vi "_PC_SaveFile exportDocData.vi"(7 "xy graph ref":refnum<vi>, 8 "error in (no error)":errorcluster) -> (0 "error out":errorcluster)   [LabVIEW 2018]
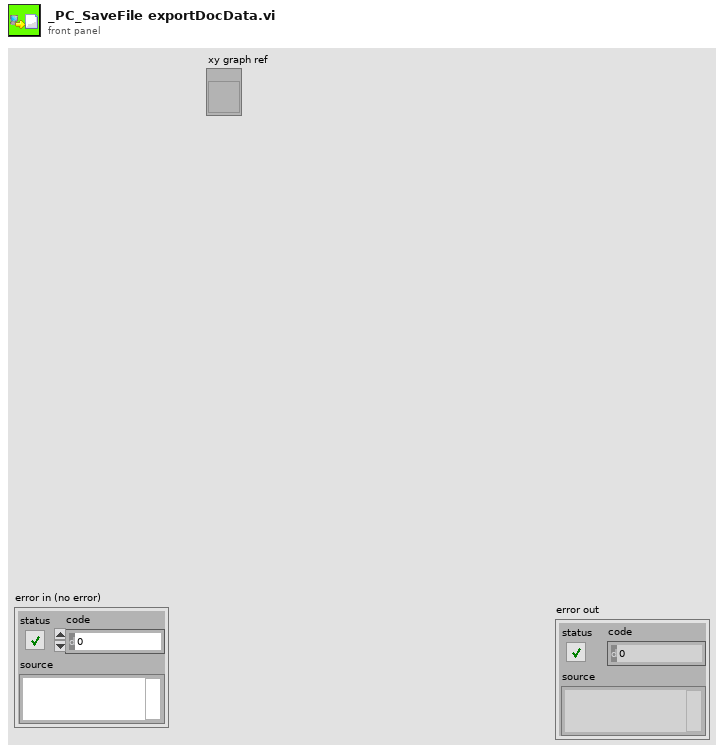
[diagram p1: front panel]
types:
  T1 = enum16{"open", "replace", "create", "open or create", "replace or create", "replace or create with confirmation"}
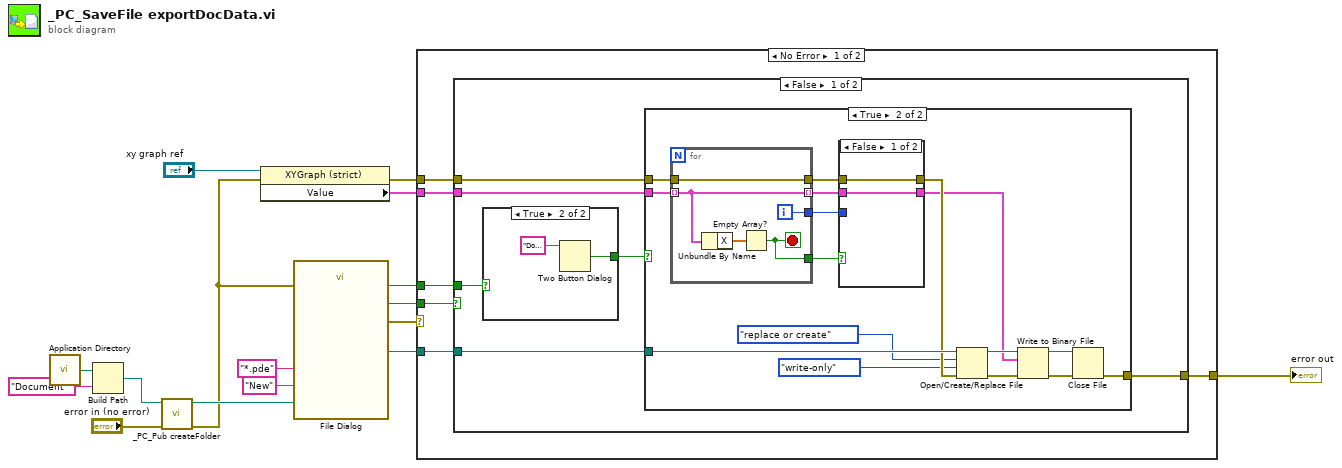
[diagram p0: block diagram]
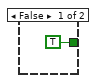
[diagram p2: hidden frame]
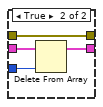
[diagram p4: hidden frame]
diagram:
  n1 = call <vilib>:"Application Directory.vi"() -> ("Application Directory"=w10:path)
  n2 = Build Path(base path=w10, name or relative path="Document") -> (appended path=w4:path)
  n3 = call "_PC_Pub createFolder.vi"("error in (no error)"="error in (no error)", "path (use dialog)"=w4) -> ("error out"=w1:errorcluster, "created path"=w2:path)  [unwired: 8 in]
  n4 = property class="XYGraph (strict)"(reference="xy graph ref", error in=w1) -> (error out=w14:errorcluster, "Value"=w15:cluster{"X":dbl[], "Y":sgl[]}[])  [unwired: 1 out]
  n5 = call "File Dialog"("start path"=w2, "default name"="New", "error in"=w1, "pattern (all files)"="*.pde") -> ("selected path"=w8:path, "exists"=w6:bool, "cancelled"=w7:bool, "error out"=w5:errorcluster)  [unwired: 8 in]
  n6 = case shown="No Error" w5 {
    selector: w5 -> [_ w61]
    tunnel: w15 -> [w22 _]
    tunnel: w14 -> [w21 _]
    tunnel: [w20 w61] -> w13
    tunnel: w8 -> [w19 _]
    tunnel: w7 -> [w18 _]
    tunnel: w6 -> [w17 _]
    frame No Error {
      n7 = case shown="False" w18 {
        tunnel: w22 -> [w28 _]
        tunnel: w21 -> [w27 w60]
        tunnel: w17 -> [w26 _]
        tunnel: w19 -> [w24 _]
        tunnel: [w23 w60] -> w20
        frame False {
          n8 = case shown="True" w26 {
            tunnel: [TRUE ("T button?") w30] -> w25
            frame False {
            }
            frame True {
              n9 = Two Button Dialog(message="Do you want overwrite this file?") -> (T button?=w30:bool)  [unwired: 2 in]
            }
          }
          n10 = case shown="True" w25 {
            tunnel: w28 -> [_ w42]
            tunnel: w27 -> [w32 w41]
            tunnel: w24 -> [_ w44]
            tunnel: [w32 w43] -> w23
            frame False {
            }
            frame True {
              n11 = for {
                tunnel: w42 -> [w58] mode=indexing
                tunnel: w41 -> [w57]
                tunnel: [w58] -> w38 mode=indexing
                tunnel: [w57] -> w37
                tunnel: [w56] -> w40
                tunnel: [w55] -> w39
                i -> [w55]
                stop <- w56 stop-if-true
                n12 = Unbundle By Name(w58) -> ("X"=w59:dbl[])
                n13 = Empty Array?(array=w59) -> (empty?=w56:bool)
              }
              n14 = case shown="False" w40 {
                tunnel: w39 -> [_ w53]
                tunnel: w38 -> [w50 w54]
                tunnel: w37 -> [w49 w51]
                tunnel: [w50 w52] -> w35
                tunnel: [w49 w51] -> w36
                frame False {
                }
                frame True {
                  n15 = Delete From Array(array=w54, index=w53) -> (array with subset deleted=w52:cluster{"X":dbl[], "Y":sgl[]}[])  [unwired: 1 in, 1 out]
                }
              }
              n16 = Open/Create/Replace File(file path (use dialog)=w44, error in=w36, operation (0:open)=T1."replace or create", access (0:read/write)=enum16{"read/write", "read-only", "write-only"}."write-only") -> (refnum out=w46:refnum<file>, error out=w45:errorcluster)  [unwired: 2 in, 1 out]
              n17 = Write to Binary File(file (use dialog)=w46, data=w35, error in=w45) -> (refnum out=w48:refnum<file>, error out=w47:errorcluster)  [unwired: 3 in, 1 out]
              n18 = Close File(refnum=w48, error in=w47) -> (error out=w43:errorcluster)  [unwired: 1 out]
            }
          }
        }
        frame True {
        }
      }
    }
    frame Error {
    }
  }
  "error out" <- w13
